vi "LEBITplc.ProcConstructor.vi"(0 "i ref in":refnum<vi>, 5 "error in(no error)":errorcluster) -> (14 "i ref out":refnum<vi>, 19 "error out":errorcluster)   [LabVIEW 2014, in "LEBITplc.lvlib"]
doc: "This is the constructor of a class.\n\nLicense Agreement for this software:\n\nCopyright (C)\nGesellschaft für Schwerionenforschung, GSI\nPlanckstr. 1\n64291 Darmstadt\nGermany\n\nContact: D.Beck@gsi.de \n\nThis program is free software; you can redistribute it and/or modify it under the terms of the \nGNU General Public License as published by the Free Software Foundation; either version 2 of \nthe license, or (at your option) any later version.\n\nThis program is distributed in the hope that it will be useful, but WITHOUT ANY WARRANTY; \nwithout even the implied warranty of MERCHANTABILITY or FITNESS FOR A PARTICULAR PURPOSE. See the GNU General License for more details (http://www.gnu.org).\n\nGesellschaft für Schwerionenforschung, GSI\nPlanckstr. 1, 64291 Darmstadt, Germany\nFor all questions and ideas contact: M.Richter@gsi.de, H.Brand@gsi.de or D.Beck@gsi.de.\nLast update: 16-JUN-2004"
uses:
  LEBITplc.lvlib
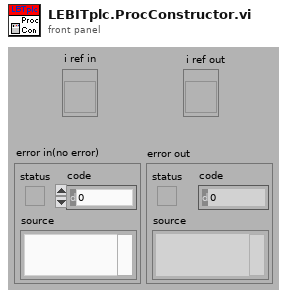
[diagram p1: front panel]
types:
  T1 = typedef "LEBITplc.lvlib/LEBITplc.i attribute.ctl" = cluster{"LLFLocation":string, "SetFileLocation":string, "nickNames":string[], "setValuePLCServiceID":i32[], "GUIServiceID":i32[], "monValuePLC":string[], "SetValueServiceID":i32[], "MonValueServiceID":i32[], "SetValue":dbl[][], "SetValueMin":dbl[], "SetValueMax":dbl[], "SetValueInfoServiceID":i32[], "GUINames":string[], "ListOfBases":string[], "Scale":dbl[], "Offset":dbl[], "setValuePLC":string[], "BaseName":string[], "ScaleServiceID":i32[], "OffsetServiceID":i32[], "AllPLCValues":string[], "CondSpecialArray":string[][], "CondSpecialIndex":i32[], "CondSpecialMonValue":dbl[], "RecentlyChanged":i32[], "SetFileLocationID":i32, "Dependent-Monitors":string[][], "LastLoadedFiles":string[], "IonGuideCalibLocation":string, "Monitor Dependent":string[], "Special":string[], "PLC?":bool[], "Start Date":string, "ListOfBasesServiceID":i32, "SETRA VISA resource":refnum<visa-resource-name>}
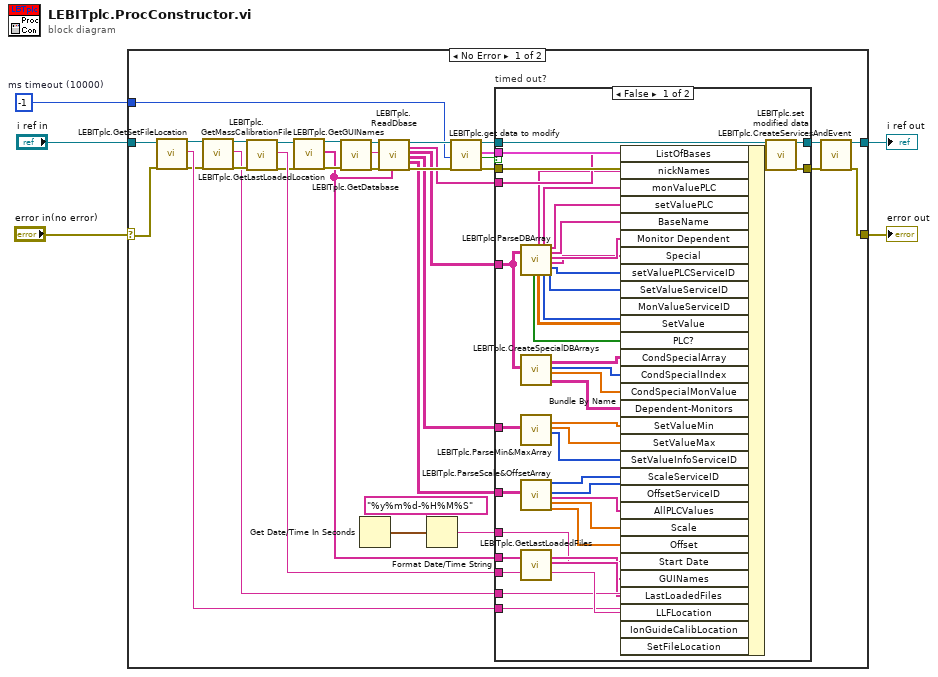
[diagram p0: block diagram]
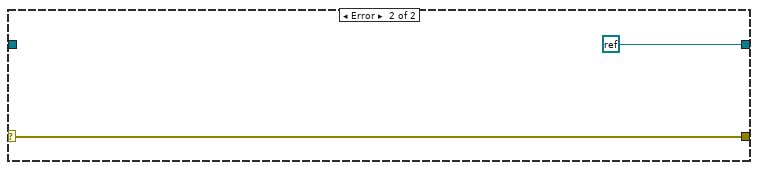
[diagram p3: hidden frame]
diagram:
  w1 = -1  # ms timeout (10000)
  n1 = case shown="No Error" "error in(no error)" {
    selector: "error in(no error)" -> [w18 w85]
    tunnel: [w26 w85] -> w5
    tunnel: "i ref in" -> [w19 _]
    tunnel: [w27 refnum<k0> refnum] -> w2
    tunnel: w1 -> [w30 _]
    frame No Error {
      n2 = call "LEBITplc.GetSetFileLocation.vi"("i ref in"=w19, "error in (no error)"=w18) -> ("i ref out"=w13:refnum<vi>, "SetFilelLocation"=w17:string, "error out"=w10:errorcluster)  [unwired: 15 in]
      n3 = call "LEBITplc.GetMassCalibrationFile.vi"("i ref in"=w13, "error in (no error)"=w10) -> ("i ref out"=w12:refnum<vi>, "SetFilelLocation"=w9:string, "error out"=w11:errorcluster)  [unwired: 15 in]
      n4 = call "LEBITplc.GetLastLoadedLocation.vi"("i ref in"=w12, "error in (no error)"=w11) -> ("i ref out"=w16:refnum<vi>, "LLFLocation"=w15:string, "error out"=w14:errorcluster)  [unwired: 15 in]
      n5 = call "LEBITplc.GetGUINames.vi"("i ref in"=w16, "error in (no error)"=w14) -> ("i ref out"=w22:refnum<vi>, "GUINames"=w20:string[], "error out"=w21:errorcluster)  [unwired: 15 in]
      n6 = call "LEBITplc.GetDatabase.vi"("i ref in"=w22, "error in (no error)"=w21) -> ("i ref out"=w36:refnum<vi>, "database"=w38:string, "error out 2"=w39:errorcluster)  [unwired: 15 in]
      n7 = Get Date/Time In Seconds() -> (seconds since 1Jan1904=w8:timestamp)
      n8 = call "LEBITplc.ReadDbase.vi"("i ref in"=w36, "Data Source"=w38, "error in (no error)"=w39, "Associated Panels"=w20) -> ("i ref out"=w35:refnum<vi>, "ListOfBases"=w24:string[], "DBArray"=w31:string[][], "Min&MaxArray"=w25:string[][], "Scale And Offset Array"=w23:string[][], "error out"=w37:errorcluster)  [unwired: 10 in]
      n9 = Format Date/Time String(time format string (%c)="%y%m%d-%H%M%S", seconds (now)=w8) -> (date/time string=w7:string)  [unwired: 1 in]
      n10 = call "LEBITplc.get data to modify.vi"("i ref in"=w35, "ms timeout (10000)"=w30, "error in (no error)"=w37) -> ("i ref out"=w33:refnum<vi>, "i attribute"=w40:T1, "timed out"=w34:bool, "error out"=w32:errorcluster)  [unwired: 13 in]
      n11 = case "timed out?" shown="False" w34 {
        tunnel: w40 -> [w78 _]
        tunnel: w33 -> [w79 w83]
        tunnel: [w81 w83] -> w29
        tunnel: [w80 w82] -> w28
        tunnel: w32 -> [w74 w82]
        tunnel: w31 -> [w59 _]
        tunnel: w25 -> [w60 _]
        tunnel: w24 -> [w73 _]
        tunnel: w23 -> [w72 _]
        tunnel: w15 -> [w55 _]
        tunnel: w17 -> [w52 _]
        tunnel: w20 -> [w54 _]
        tunnel: w9 -> [w51 _]
        tunnel: w7 -> [w41 _]
        frame False {
          n12 = call "LEBITplc.ParseDBArray.vi"("DBArray"=w59) -> ("PLC?"=w43:bool[], "nickname"=w67:string[], "SetValue"=w61:dbl[][], "monValuePLC"=w77:string[], "MonValueServiceID"=w62:i32[], "setValuePLC"=w76:string[], "BaseNames"=w48:string[], "MonitorDependent"=w47:string[], "Special"=w45:string[], "setValuePLCServiceID"=w46:i32[], "SetValueServiceID"=w63:i32[])  [unwired: 8 in]
          n13 = call "LEBITplc.CreateSpecialDBArrays.vi"("DBArray"=w59) -> ("CondSpecialArray"=w44:string[][], "CondSpecialIndex"=w58:i32[], "CondSpecialMonValue"=w57:dbl[], "Dependent Monitors"=w56:string[][])  [unwired: 15 in]
          n14 = call "LEBITplc.ParseMin&MaxArray.vi"("Min&MaxArray"=w60) -> ("MinSetValue"=w66:dbl[], "MaxSetValue"=w65:dbl[], "SetValueInfoServiceId"=w64:i32[])  [unwired: 16 in]
          n15 = call "LEBITplc.ParseScale&OffsetArray.vi"("ScaleAndOffsetArray"=w72) -> ("ScaleServicesID"=w68:i32[], "OffsetServicesID"=w69:i32[], "AllPLCValues"=w50:string[], "Scale"=w70:dbl[], "Offset"=w71:dbl[])  [unwired: 14 in]
          n16 = call "LEBITplc.GetLastLoadedFiles.vi"("GUINames"=w54, "LLFLocation"=w55) -> ("GUINames"=w42:string[], "Last Loaded File Array"=w49:string[], "LLFLocation"=w53:string)  [unwired: 15 in]
          n17 = Bundle By Name(cluster=w78, "ListOfBases"=w73, "nickNames"=w67, "monValuePLC"=w77, "setValuePLC"=w76, "BaseName"=w48, "Monitor Dependent"=w47, "Special"=w45, "setValuePLCServiceID"=w46, "SetValueServiceID"=w63, "MonValueServiceID"=w62, "SetValue"=w61, "PLC?"=w43, "CondSpecialArray"=w44, "CondSpecialIndex"=w58, "CondSpecialMonValue"=w57, "Dependent-Monitors"=w56, "SetValueMin"=w66, "SetValueMax"=w65, "SetValueInfoServiceID"=w64, "ScaleServiceID"=w68, "OffsetServiceID"=w69, "AllPLCValues"=w50, "Scale"=w70, "Offset"=w71, "Start Date"=w41, "GUINames"=w42, "LastLoadedFiles"=w49, "LLFLocation"=w53, "IonGuideCalibLocation"=w51, "SetFileLocation"=w52) -> (w75:T1)
          n18 = call "LEBITplc.set modified data.vi"("i ref in"=w79, "i attribute"=w75, "error in (no error)"=w74) -> ("i ref out"=w81:refnum<vi>, "error out"=w80:errorcluster)  [unwired: 15 in]
        }
        frame True {
        }
      }
      n19 = call "LEBITplc.CreateServicesAndEvent.vi"("i ref in"=w29, "error in(no error)"=w28) -> ("i ref out"=w27:refnum<vi>, "error out"=w26:errorcluster)  [unwired: 16 in]
    }
    frame Error {
    }
  }
  "i ref out" <- w2
  "error out" <- w5
